vi "AutoChop.vi"(6 "Points to chop off the bottom edge":i32, 7 "Points to chop off the top edge":i32, 10 "use auto chop":bool, 11 "Intensity InfoOUT":cluster{dbl[], dbl[]}[](array[cluster])) -> (3 "Intensity InfoOUT 2":cluster{dbl[], dbl[]}[](array[cluster]))   [LabVIEW 2016]
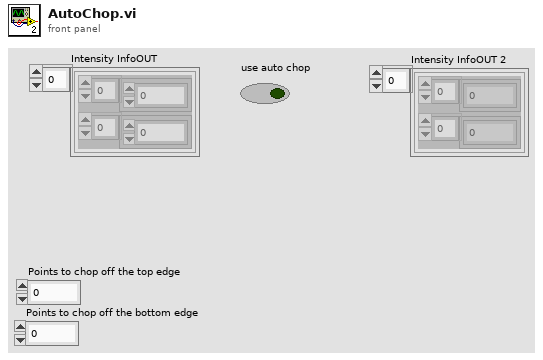
[diagram p1: front panel]
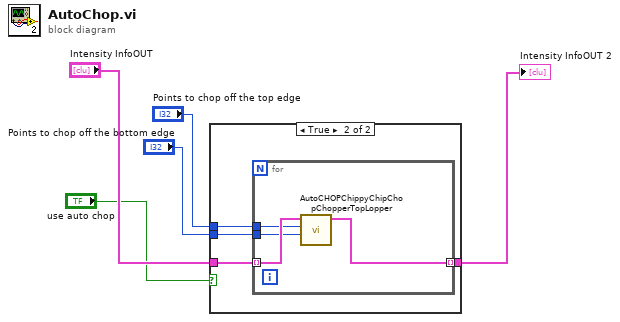
[diagram p0: block diagram]
diagram:
  n1 = case shown="True" "use auto chop" {
    tunnel: "Intensity InfoOUT" -> [w6 w10]
    tunnel: [w6 w9] -> w4
    tunnel: "Points to chop off the top edge" -> [_ w8]
    tunnel: "Points to chop off the bottom edge" -> [_ w7]
    frame False {
    }
    frame True {
      n2 = for {
        tunnel: w10 -> [w14] mode=indexing
        tunnel: [w13] -> w9 mode=indexing
        tunnel: w8 -> [w12]
        tunnel: w7 -> [w11]
        n3 = call "AutoCHOPChippyChipChopChopperTopLopper.vi"("Points to chop off the bottom edge"=w11, "Points to chop off the top edge"=w12, "Vsrc and Current In"=w14) -> ("Vsrc and Current Out"=w13:cluster{dbl[], dbl[]})  [unwired: 8 in]
      }
    }
  }
  "Intensity InfoOUT 2" <- w4
